vi "ClearCOM.vi"(8 "error in (no error)":errorcluster, 11 "Data In":T1) -> (0 "error out":errorcluster, 3 "Data out":T1)   [LabVIEW 2014]
uses:
  controls/Data1.ctl
  controls/Payjson.ctl
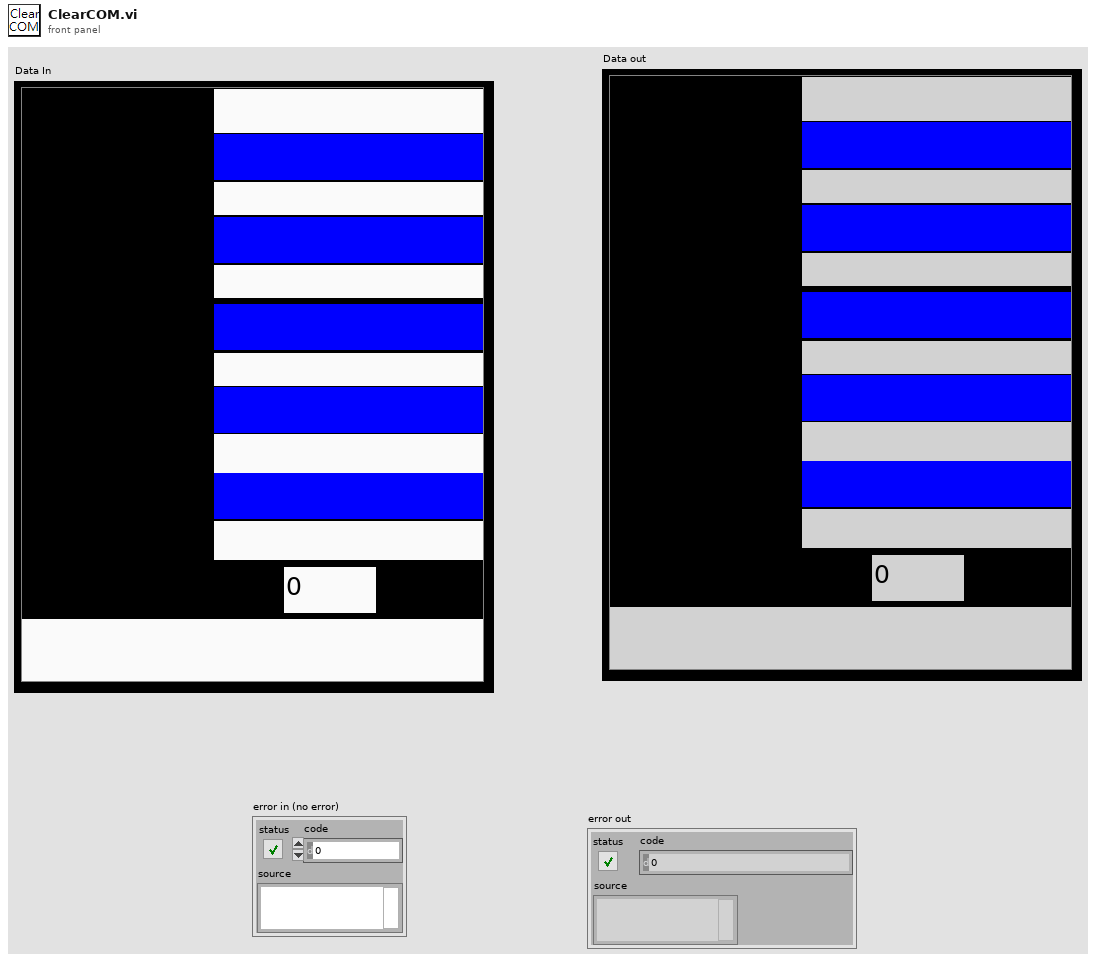
[diagram p1: front panel]
types:
  T1 = typedef "Data1.ctl" = cluster{"Date":string, "BarCode1":string, "BarCode2":string, "BarCode3":string, "Message":string, "OK Count":u16, "NG Count":u16, "Total Count":u16, "ModelData":string[][], "OK&NG":bool, "COM1":refnum<visa-resource-name>, "COM2":refnum<visa-resource-name>, "IO":i32, "Time":u32, "TCP":refnum<k5>, "TCP 2":refnum<k5>, "COM1 2":refnum<visa-resource-name>, "CheckNum":string, "BarCode1_1":string, "BarCode2_1":string, "BarCode3_1":string, "日期":string, "機種":string, "機號":string, "商品條碼1":string, "OK_1":string, "OK":string, "NG":string, "NG_1":string, "Total":string, "Total_1":string, "ClaerTime":u32, "Pjson":T2, "LotNo":string[], "CheckParsArray":string[], "BarCode4":string, "BarCode4_1":string, "商品條碼2":string, "BarCode5":string, "BarCode5_1":string, "商品條碼3":string, "ReScanNG":i32, "NGTimeCT":u32}
  T2 = typedef "Payjson.ctl" = cluster{"DEPT":string, "LINE":string, "STANO":string, "WORKNO":string, "PRODSN":string, "COMPNTID":string, "COMPNTLOT":string, "COMPNTSN":string, "USEDQTY":i16, "OPDATE":string, "OPUSER":string, "RECVDATE":string, "MMODU":string}[]
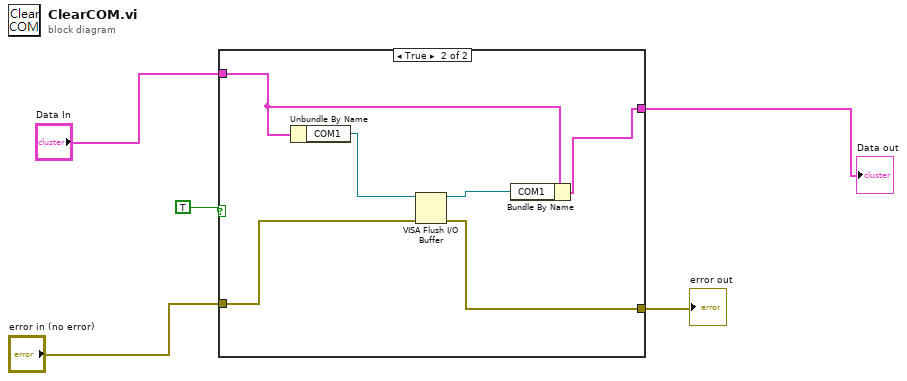
[diagram p0: block diagram]
diagram:
  n1 = case shown="True" TRUE {
    tunnel: [w6 w11] -> w1
    tunnel: "error in (no error)" -> [w7 w9]
    tunnel: [w7 w8] -> w4
    tunnel: "Data In" -> [w6 w12]
    frame False {
    }
    frame True {
      n2 = Unbundle By Name(w12) -> ("COM1"=w13:refnum<visa-resource-name>)
      n3 = VISA Flush I/O Buffer(VISA resource name=w13, error in (no error)=w9) -> (VISA resource name out=w10:refnum<visa-resource-name>, error out=w8:errorcluster)  [unwired: 1 in]
      n4 = Bundle By Name(cluster=w12, "COM1"=w10) -> (w11:T1)
    }
  }
  "error out" <- w4
  "Data out" <- w1
